vi "Flatten UIP Value.vi"(11 "ValueUIP In":refnum<class "ValueUIP.lvclass">) -> (0 "Error Out":errorcluster, 2 "String Value":string, 3 "ValueUIP Out":refnum<class "ValueUIP.lvclass">)   [LabVIEW 2015, in "ValueUIP.lvclass"]
doc: "Overwrite this abstract method to implement child behavior for flattening the UIP private data into XML compatible string format."
uses:
  ValueUIP.lvclass
  ValueUIP.lvclass/ValueUIP.ctl
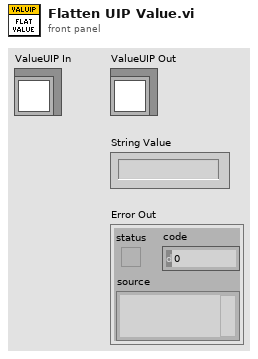
[diagram p1: front panel]
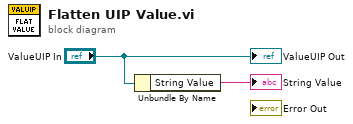
[diagram p0: block diagram]
diagram:
  n1 = Unbundle By Name("ValueUIP In") -> ("String Value"=→"String Value":string)
  "ValueUIP Out" <- "ValueUIP In"
